vi "set_material_parameters_subset.vi"(8 "error in (no error)":errorcluster, 9 "Material number":u8, 10 "Cluster Controls[]":refnum<vi>[](array[refnum]), 11 "VISA resource name":refnum<visa-resource-name>) -> (0 "error out":errorcluster, 3 "VISA Refnum out":refnum<visa-resource-name>)   [LabVIEW 2018]
uses:
  Low Level/material_parameter_ring.ctl
panel:
  out "Label.Text":string
  in  "Material parameter":T1 items=["Density (g/cc)", "Z-Ratio", "Master Tooling (%)", "Control Loop", "Process Gain (A/s/%)", "Time Constant (s)", "Dead Time (s)", "Source", "Maximum Power (%)", "Minimum Power (%)", "Max Power Option", "PreCond Soak Power (%)", "PreCond Rise Time (s) (mm:ss)", "PreCond Soak Time (s) (mm:ss)", "Soak Power 1 (%)", "Rise Time 1 (s) (mm:ss)", "Soak Time 1 (s) (mm:ss)", "Soak Power 2 (%)", "Rise Time 2 (s) (mm:ss)", "Soak Time 2 (s) (mm:ss)", "Auto Soak 2", "Dep After Pre-Dep", "Delay Option", "Control Delay Time (s) (mm:ss)", "Shutter Delay Accur (%)", "Transfer Sensor", "Transfer Tooling (%)", "Feed Power (%)", "Feed Ramp Time (s) (mm:ss)", "Feed Time (s) (mm:ss)", "Idle Power (%)", "Idle Ramp Time (s) (mm:ss)", "Rate (A/s)", "Time Limit (s) (mm:ss)", "Rate Filter Time (s)", "Time Power Avg Time (minutes)", "Ion Assist Deposit", "On Final Thickness", "Ramp 1 Rate (A/s)", "Start Ramp 1 (kA)", "Ramp 1 Time (s) (mm:ss)", "Ramp 2 Rate (A/s)", "Start Ramp 2 (kA)", "Ramp 2 Time (s) (mm:ss)", "RateWatcher Option", "RateWatcher Time (s) (mm:ss)", "RateWatcher Accuracy (%)", "Multipoint", "Aggregate Multiplier", "Sensor 1 Failure Action", "Sensor 2 Failure Action", "Sensor 3 Failure Action", "Sensor 4 Failure Action", "Sensor 5 Failure Action", "Sensor 6 Failure Action", "Sensor 7 Failure Action", "Sensor 8 Failure Action", "Sensor 1 Failure Trigger", "Sensor 2 Failure Trigger", "Sensor 3 Failure Trigger", "Sensor 4 Failure Trigger", "Sensor 5 Failure Trigger", "Sensor 6 Failure Trigger", "Sensor 7 Failure Trigger", "Sensor 8 Failure Trigger", "Sensor 1 Weight (%)", "Sensor 2 Weight (%)", "Sensor 3 Weight (%)", "Sensor 4 Weight (%)", "Sensor 5 Weight (%)", "Sensor 6 Weight (%)", "Sensor 7 Weight (%)", "Sensor 8 Weight (%)", "Sensor 1 Tooling (%)", "Sensor 2 Tooling (%)", "Sensor 3 Tooling (%)", "Sensor 4 Tooling (%)", "Sensor 5 Tooling (%)", "Sensor 6 Tooling (%)", "Sensor 7 Tooling (%)", "Sensor 8 Tooling (%)", "Sensor 1 CrystalTwo Tooling (%)", "Sensor 2 CrystalTwo Tooling (%)", "Sensor 3 CrystalTwo Tooling (%)", "Sensor 4 CrystalTwo Tooling (%)", "Sensor 5 CrystalTwo Tooling (%)", "Sensor 6 CrystalTwo Tooling (%)", "Sensor 7 CrystalTwo Tooling (%)", "Sensor 8 CrystalTwo Tooling (%)", "Sensor 1 Cal Thickness (kA)", "Sensor 2 Cal Thickness (kA)", "Sensor 3 Cal Thickness (kA)", "Sensor 4 Cal Thickness (kA)", "Sensor 5 Cal Thickness (kA)", "Sensor 6 Cal Thickness (kA)", "Sensor 7 Cal Thickness (kA)", "Sensor 8 Cal Thickness (kA)", "Sensor 1 Xtal Position First", "Sensor 2 Xtal Position First", "Sensor 3 Xtal Position First", "Sensor 4 Xtal Position First", "Sensor 5 Xtal Position First", "Sensor 6 Xtal Position First", "Sensor 7 Xtal Position First", "Sensor 8 Xtal Position First", "Sensor 1 Xtal Position Last", "Sensor 2 Xtal Position Last", "Sensor 3 Xtal Position Last", "Sensor 4 Xtal Position Last", "Sensor 5 Xtal Position Last", "Sensor 6 Xtal Position Last", "Sensor 7 Xtal Position Last", "Sensor 8 Xtal Position Last", "Sensor", "Failure Action", "CrystalTwo Tooling (%)", "Xtal Position First", "Xtal Position Last", "Backup Sensor", "Backup Tooling (%)", "Quality Percent (%)", "Quality Counts", "Stability Single (Hz)", "Stability Total (Hz)", "Recorder Output", "Recorder Function", "Recorder Range"]
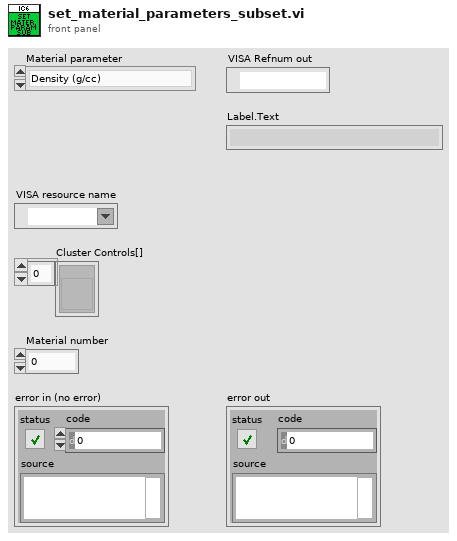
[diagram p1: front panel]
types:
  T1 = typedef "material_parameter_ring.ctl" = u16
  T2 = typedef "LVStringsAndValuesArrayTypeDef_U16.ctl" = cluster{"String":string, "Value":u16}[]
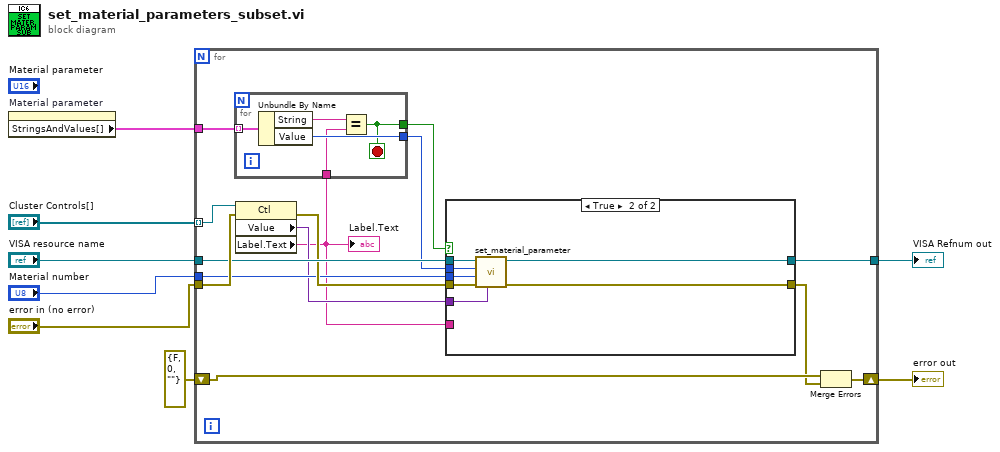
[diagram p0: block diagram]
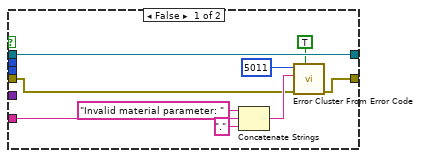
[diagram p2: hidden frame]
diagram:
  n1 = property on="Material parameter" class="Ring (strict)"() -> ("StringsAndValues[]"=w3:T2)  [unwired: 2 in, 2 out]
  n2 = for {
    tunnel: "VISA resource name" -> [w20]
    tunnel: [w17] -> w5
    tunnel: "Material number" -> [w18]
    tunnel: w3 -> [w15]
    tunnel: "Cluster Controls[]" -> [w22] mode=indexing
    tunnel: "error in (no error)" -> [w21]
    shift-right: [w13] -> w2
    shift-left: errorcluster {"status"=FALSE, "code"=0, "source"=""} ("error IO") -> [w12]
    n3 = property class="Ctl"(reference=w22, error in=w21) -> (error out=w19:errorcluster, "Value"=w16:variant, "Label.Text"=w14:string)  [unwired: 1 out]
    "Label.Text" <- w14
    n4 = for {
      tunnel: [w43] -> w9
      tunnel: w15 -> [w42] mode=indexing
      tunnel: w14 -> [w40]
      tunnel: [w39] -> w10
      stop <- w39 stop-if-true
      n5 = Unbundle By Name(w42) -> ("String"=w41:string, "Value"=w43:u16)
      n6 = Equal?(x=w41, y=w40) -> (x = y?=w39:bool)
    }
    n7 = case shown="True" w10 {
      tunnel: w20 -> [w31 w38]
      tunnel: w19 -> [w24 w37]
      tunnel: w18 -> [_ w36]
      tunnel: [w31 w35] -> w17
      tunnel: [w25 w34] -> w11
      tunnel: w9 -> [_ w33]
      tunnel: w16 -> [_ w32]
      tunnel: w14 -> [w23 _]
      frame False {
        n8 = Concatenate Strings("Invalid material parameter: " ("error message (\"\")"), w23, "." ("string")) -> (w26:string)
        n9 = call <vilib>:"Error Cluster From Error Code.vi"("show call chain? (False)"=TRUE, "error in (no error)"=w24, "error message (\"\")"=w26, "error code (0)"=5011) -> ("error out"=w25:errorcluster)  [unwired: 5 in]
      }
      frame True {
        n10 = call "set_material_parameter.vi"("Parameter value"=w32, "error in (no error)"=w37, "Material number"=w36, "Material parameter"=w33, "VISA resource name"=w38) -> ("error out"=w34:errorcluster, "VISA resource name out"=w35:refnum<visa-resource-name>)  [unwired: 5 in]
      }
    }
    n11 = Merge Errors(w12, w11) -> (w13:errorcluster)
  }
  "error out" <- w2
  "VISA Refnum out" <- w5
